vi "niFPGA Initial Condition_m.vi"   [LabVIEW 2017]
doc: "Produces a predefined initial condition immediately after the first time you call or initialize the VI. The data type you wire to <B>input</B> determines the <B>output</B> data type."
uses:
  <vilib>/rvi/Analysis/common/FxpNativeNode/niFpgaFxpNative.xnode
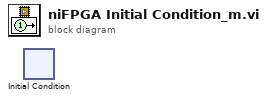
[diagram p0: block diagram]
diagram:
  n1 = xnode ("Initial Condition")() -> ()  [unwired: 3 in, 1 out]
